vi "Client.vi"() -> ()   [LabVIEW 2016]
doc: "This VI acts as a server for an incoming websockets connection. Receives/sends string data to the connected client.\nWebSockets 1.6.0.22\nSam Sharp - MediaMongrels Ltd\nCopyright (c) 2016, MediaMongrels Ltd"
uses:
  StatusCode.ctl
  WebSockets.lvlib
panel:
  out "Status Code":T1=1000 items=["Normal Closure"=1000, "Going Away"=1001, "Protocol Error"=1002, "Wrong Data Type"=1003, "Reserved 1004"=1004, "Reserved 1005"=1005, "Reserved 1006"=1006, "Non Consistent Data Type"=1007, "Policy Violation"=1008, "Message Too Big"=1009, "Extensions Negotiation Error"=1010, "Unexpected Condition"=1011, "Reserved 1015"=1015]
  out "Close Reason":string
  in  "WS URI":string="ws://localhost:6123/resource/name"
  out "Resource Name":string
  out "Request URI":string
  out "HTTP Headers":variant
  in  "Stop":bool
  out "Received Data":string
  in  "Send":bool
  in  "Data":string
  # "WebSockets Example Client"
  # "This VI is a simple example of sending/receiving data using WebSockets.\nIt opens a WebSockets connection on Port 6123 and\nthen displays incoming string data. Strings can also be sent back to the client.\n\nInstructions for use:\n1) Run the SingleConnection.vi VI\n2) Set a suitable websocket URI including a resource name matching the one defined on the server\n2) Quickly run this VI"
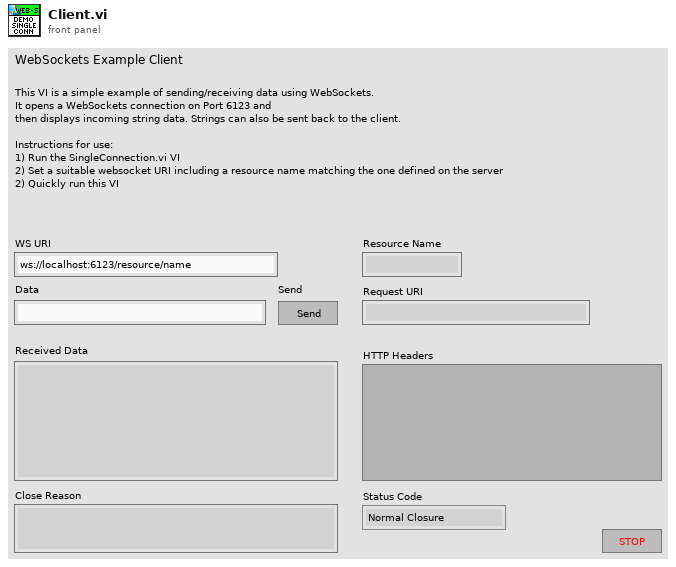
[diagram p1: front panel]
types:
  T1 = typedef "WebSockets.lvlib/StatusCode.ctl" = u16
  T2 = typedef "WebSockets.lvlib/Opcode.ctl" = enum8{"Continuation Frame", "Text Frame", "Binary Frame", "Reserved 3", "Reserved 4", "Reserved 5", "Reserved 6", "Reserved 7", "Connection Close", "Ping", "Pong", "Reserved B", "Reserved C", "Reserved D", "Reserved F"}
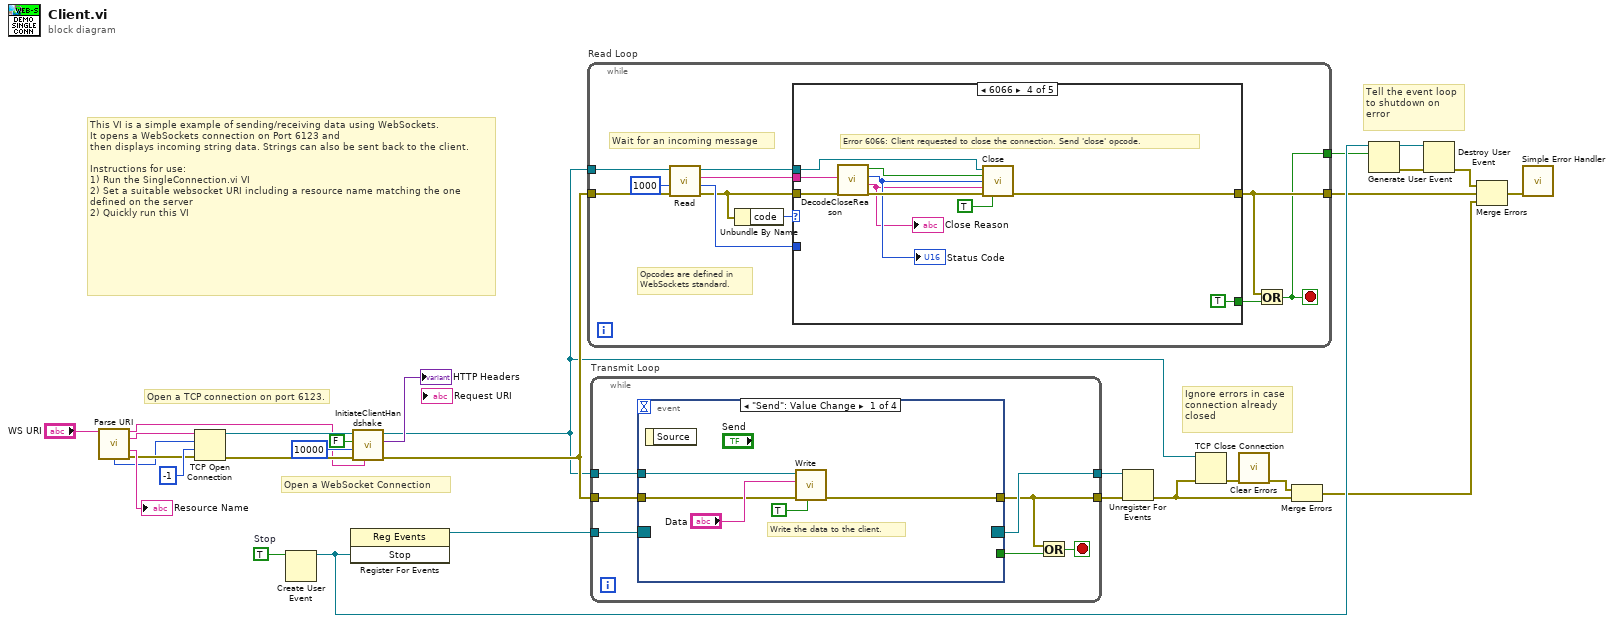
[diagram p0: block diagram]
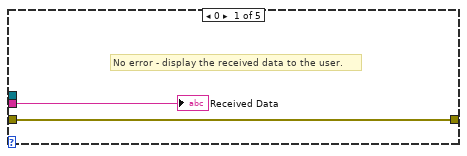
[diagram p2: hidden frame]
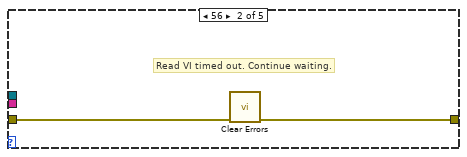
[diagram p3: hidden frame]
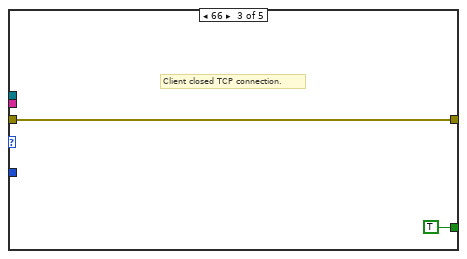
[diagram p4: hidden frame]
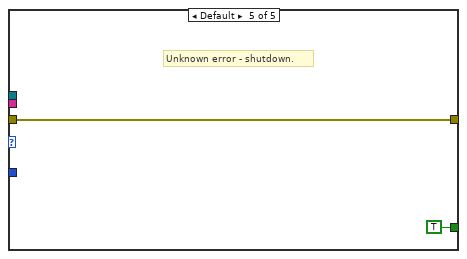
[diagram p5: hidden frame]
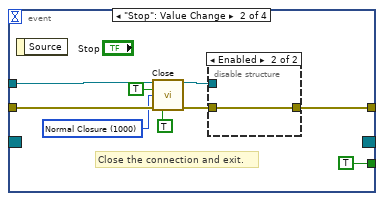
[diagram p6: hidden frame]
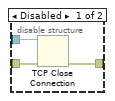
[diagram p7: hidden frame]
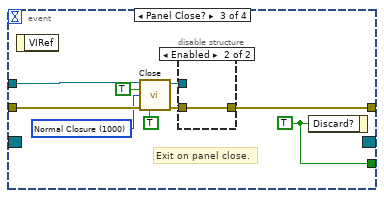
[diagram p8: hidden frame]
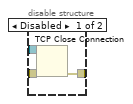
[diagram p9: hidden frame]
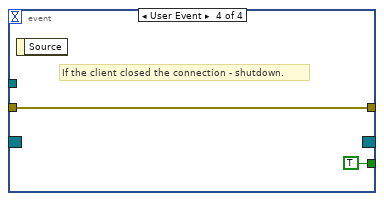
[diagram p10: hidden frame]
diagram:
  w25 = TRUE  # Stop
  # "Ignore errors in case\nconnection already\nclosed"
  # "Tell the event loop to shutdown on error"
  # "This VI is a simple example of sending/receiving data using WebSockets.\nIt opens a WebSockets connection on Port 6123 and\nthen displays incoming string data. Strings can also be sent back to the client.\n\nInstructions for use:\n1) Run the SingleConnection.vi VI\n2) Set a suitable websocket URI including a resource name matching the one defined on the server\n2) Quickly run this VI"
  # "Open a WebSocket Connection"
  # "Open a TCP connection on port 6123."
  n1 = call "Parse URI.vi"("URI"="WS URI") -> ("URI Out"=w6:string, "Hostname"=w5:string, "Resource Name"=→"Resource Name":string, "Port"=w1:u16, "error out"=w3:errorcluster)  [unwired: 8 in, 2 out]
  n2 = TCP Open Connection(address=w5, remote port or service name=w1, timeout ms (60000)=-1 ("timeout ms (25000)"), error in (no error)=w3) -> (connection ID=w28:refnum<k5>, error out=w27:errorcluster)  [unwired: 1 in]
  n3 = Create User Event(user event datatype=w25) -> (user event=w23:refnum<user-event>)  [unwired: 1 in, 1 out]
  n4 = register-events(w23) -> (reference out=w26:refnum<event-registration>)  [unwired: 2 in, 1 out]
  n5 = call "InitiateClientHandshake.vi"("WS URI"=w6, "error in (no error)"=w27, "timeout ms (5000)"=10000 ("timeout ms (25000)"), "Relative URI Request (F)"=FALSE, "WebSocket Connection in"=w28) -> ("error out"=w14:errorcluster, "Return Headers Out"=→"HTTP Headers":variant, "WebSocket Connection out"=w12:refnum<k5>)  [unwired: 4 in]
  n6 = while "Read Loop" {
    tunnel: w12 -> [w40]
    tunnel: [w30] -> w22
    tunnel: [w32] -> w13
    tunnel: w14 -> [w33]
    stop <- w30 stop-if-true
    # "Wait for an incoming message"
    # "Opcodes are defined in\nWebSockets standard."
    n7 = call "Read.vi"("error in (no error)"=w33, "timeout ms (5000)"=1000 ("timeout ms (25000)"), "WebSocket Connection in"=w40) -> ("error out"=w34:errorcluster, "Opcode out"=w35:T2, "Data"=w37:string, "WebSocket Connection out"=w36:refnum<k5>)  [unwired: 5 in]
    n8 = Unbundle By Name(w34) -> ("code"=w38:i32)
    n9 = case shown="6066" w38 {
      tunnel: w37 -> [w42 _ _ w51 _]
      tunnel: [_ _ TRUE TRUE TRUE] -> w31
      tunnel: w36 -> [_ _ _ w55 _]
      tunnel: w35 -> [_ _ _ _ _]
      tunnel: w34 -> [w41 w44 w45 w53 w56]
      tunnel: [w41 w43 w45 w52 w56] -> w32
      frame 0 {
        # "No error - display the received data to the user."
        "Received Data" <- w42
      }
      frame 56 {
        # "Read VI timed out. Continue waiting."
        n10 = call <vilib>:"Clear Errors.vi"("error in (no error)"=w44) -> ("error out"=w43:errorcluster)  [unwired: 5 in, 1 out]
      }
      frame 66 {
        # "Client closed TCP connection."
      }
      frame 6066 {
        # "Error 6066: Client requested to close the connection. Send 'close' opcode."
        n11 = call "DecodeCloseReason.vi"("Data"=w51) -> ("Reason"=w47:string, "Status Code"=w49:T1, "Close Reason Given"=w50:bool)  [unwired: 8 in]
        "Close Reason" <- w47
        "Status Code" <- w49
        n12 = call "Close.vi"("WebSocket Connection in"=w55, "Send Reason (F)"=w50, "Status Code"=w49, "Reason"=w47, "error in (no error)"=w53, "Mask payload?"=TRUE) -> ("error out"=w52:errorcluster)  [unwired: 8 in, 1 out]
      }
      frame Default {
        # "Unknown error - shutdown."
      }
    }
    n13 = Or(x=w32, y=w31) -> (x .or. y?=w30:bool)
  }
  n14 = while "Transmit Loop" {
    tunnel: w12 -> [w64]
    tunnel: w26 -> [w63]
    tunnel: [w62] -> w24
    tunnel: [w58] -> w15
    tunnel: w14 -> [w61]
    stop <- w59 stop-if-true
    n15 = event shown="[0] \"Send\": Value Change" {
      selector: w63 -> [_ _ _ _]
      dyn-events: [_ _ _ _] -> w62
      timeout: _ -> [_ _ _ _]
      tunnel: w64 -> [w69 w77 w91 _]
      tunnel: [_ TRUE w89 TRUE] -> w60
      tunnel: [w66 w75 w87 w96] -> w58
      tunnel: w61 -> [w67 w73 w86 w96]
      event "Send": Value Change {
        # "Write the data to the client."
        n16 = event-data() -> ()  [unwired: 1 in, 1 out]
        n17 = call "Write.vi"("Mask payload?"=TRUE, "error in (no error)"=w67, "Data"="Data", "WebSocket Connection in"=w69) -> ("error out"=w66:errorcluster)  [unwired: 6 in, 1 out]
      }
      event "Stop": Value Change {
        w71 = T1 1000 items=["Normal Closure"=1000, "Going Away"=1001, "Protocol Error"=1002, "Wrong Data Type"=1003, "Reserved 1004"=1004, "Reserved 1005"=1005, "Reserved 1006"=1006, "Non Consistent Data Type"=1007, "Policy Violation"=1008, "Message Too Big"=1009, "Extensions Negotiation Error"=1010, "Unexpected Condition"=1011, "Reserved 1015"=1015] ("Status Code")
        # "Close the connection and exit."
        n18 = event-data() -> ()  [unwired: 1 in, 1 out]
        n19 = call "Close.vi"("WebSocket Connection in"=w77, "Send Reason (F)"=TRUE, "Status Code"=w71, "error in (no error)"=w73, "Mask payload?"=TRUE) -> ("WebSocket Connection in"=w76:refnum<k5>, "error out"=w74:errorcluster)  [unwired: 9 in]
        n20 = disable-structure shown="Enabled" {
          disable-tunnel: w76 -> [w81 _]
          disable-tunnel: [w80 w82] -> w75
          disable-tunnel: w74 -> [w79 w82]
          frame Disabled {
            n21 = TCP Close Connection(connection ID=w81, error in (no error)=w79) -> (error out=w80:errorcluster)  [unwired: 1 in, 1 out]
          }
          frame Enabled {
          }
        }
      }
      event Panel Close? {
        w84 = T1 1000 items=["Normal Closure"=1000, "Going Away"=1001, "Protocol Error"=1002, "Wrong Data Type"=1003, "Reserved 1004"=1004, "Reserved 1005"=1005, "Reserved 1006"=1006, "Non Consistent Data Type"=1007, "Policy Violation"=1008, "Message Too Big"=1009, "Extensions Negotiation Error"=1010, "Unexpected Condition"=1011, "Reserved 1015"=1015] ("Status Code")
        w89 = TRUE ("Discard?")
        # "Exit on panel close."
        n22 = event-data() -> ()  [unwired: 1 in, 1 out]
        n23 = call "Close.vi"("WebSocket Connection in"=w91, "Send Reason (F)"=TRUE, "Status Code"=w84, "error in (no error)"=w86, "Mask payload?"=TRUE) -> ("WebSocket Connection in"=w90:refnum<k5>, "error out"=w88:errorcluster)  [unwired: 9 in]
        n24 = disable-structure shown="Enabled" {
          disable-tunnel: w90 -> [w94 _]
          disable-tunnel: w88 -> [w93 w95]
          disable-tunnel: [w92 w95] -> w87
          frame Disabled {
            n25 = TCP Close Connection(connection ID=w94, error in (no error)=w93) -> (error out=w92:errorcluster)  [unwired: 1 in, 1 out]
          }
          frame Enabled {
          }
        }
        n26 = event-data("Discard?"=w89) -> ()  [unwired: 1 in, 1 out]
      }
      event User Event {
        # "If the client closed the connection - shutdown."
        n27 = event-data() -> ()  [unwired: 1 in, 1 out]
      }
    }
    n28 = Or(x=w58, y=w60) -> (x .or. y?=w59:bool)
  }
  n29 = Unregister For Events(event registration refnum=w24, error in=w15) -> (error out=w10:errorcluster)
  n30 = TCP Close Connection(connection ID=w12, error in (no error)=w10) -> (error out=w11:errorcluster)  [unwired: 1 in, 1 out]
  n31 = call <vilib>:"Clear Errors.vi"("error in (no error)"=w11) -> ("error out"=w8:errorcluster)  [unwired: 5 in, 1 out]
  n32 = Merge Errors(w8, w10) -> (w9:errorcluster)
  n33 = Generate User Event(user event=w23, event data cluster=w22) -> (user event out=w21:refnum<user-event>, error out=w20:errorcluster)  [unwired: 2 in]
  n34 = Destroy User Event(user event=w21, error in=w20) -> (error out=w19:errorcluster)
  n35 = Merge Errors(w19, w13, w9) -> (w16:errorcluster)
  n36 = call <vilib>:"Simple Error Handler.vi"("error in (no error)"=w16) -> ()  [unwired: 4 in, 5 out]
